vi "Check_Traverse_move.vi"(0 "Current position":dbl[](array[numeric])=[0.0, 0.0, 0.0] format="%.2f", 1 "Traverse Name":string, 2 "Full Check":bool, 5 "New Position":dbl[](array[numeric])=[0.0, 0.0, 0.0] format="%.2f", 7 "Model       Roll      Pitch       Yaw (deg)":dbl[](array[numeric]) format="%#.2f", 9 "Probe Volume":T2=[{"Max"=15.0, "Min"=-15.0}, {"Max"=250.0, "Min"=0.0}, {"Max"=15.0, "Min"=-15.0}] {"Min" format="%#.1f"; "Max" format="%#.1f"}, 11 "Entire Space":T2=[{"Max"=15001.0, "Min"=12000.0}, {"Max"=1000.0, "Min"=-1000.0}, {"Max"=700.0, "Min"=0.0}] {"Min" format="%#.1f"; "Max" format="%#.1f"}, 12 "Exclude Array":T1[](array[typedef])=[{"Sizes"=[{"Max"=15000.0, "Min"=0.0}, {"Max"=1000.0, "Min"=-1000.0}, {"Max"=300.0, "Min"=0.0}], "Name"="Roughness Elements", "Exclude Type"=enum."Allow only vertical moves"}, {"Sizes"=[{"Max"=17000.0, "Min"=16000.0}, {"Max"=200.0, "Min"=-200.0}, {"Max"=-50.0, "Min"=-250.0}], "Name"="B204", "Exclude Type"=enum."Exclude completely"}] {"Sizes"."Min" format="%#.1f"; "Sizes"."Max" format="%#.1f"}) -> (6 "Position At Crash":dbl[](array[numeric]) format="%.2f", 10 "Steps":dbl[][](array[numeric]) format="%.2f", 15 "Error Comments":string)   [LabVIEW 2011]
uses:
  Box_size.ctl
  Exclude_cluster.ctl
  Exclusion_type.ctl
panel:
  # "X                Y                   Z"
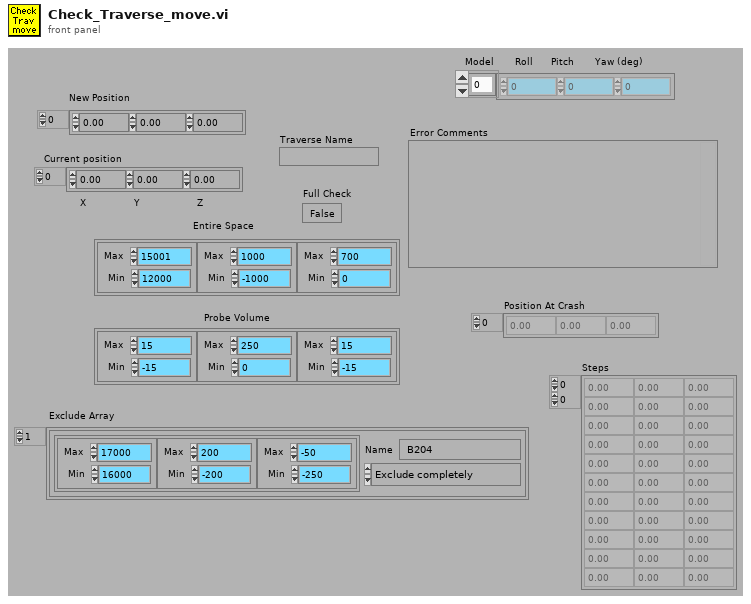
[diagram p1: front panel]
types:
  T1 = typedef "Exclude_cluster.ctl" = cluster{"Sizes":T2, "Name":string, "Exclude Type":T3}
  T2 = typedef "Box_size.ctl" = cluster{"Max":dbl, "Min":dbl}[]
  T3 = typedef "Exclusion_type.ctl" = enum16{"Exclude completely", "Allow only vertical moves"}
  T4 = enum16{"To Traverse Coordinates", "To User Coordinates"}
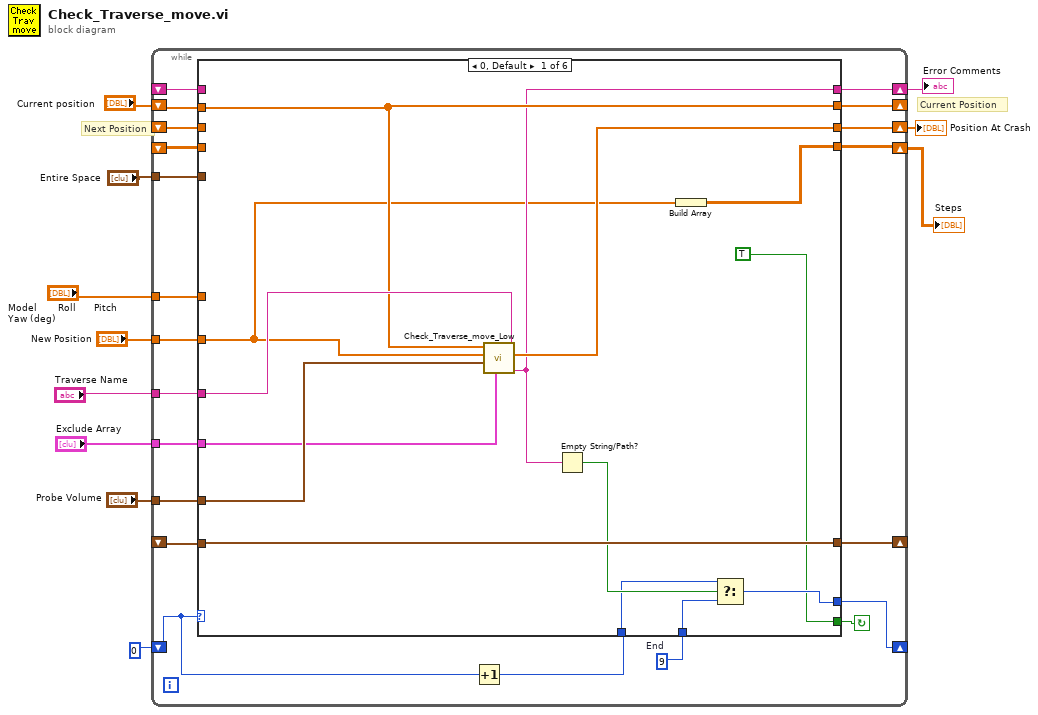
[diagram p0: block diagram]
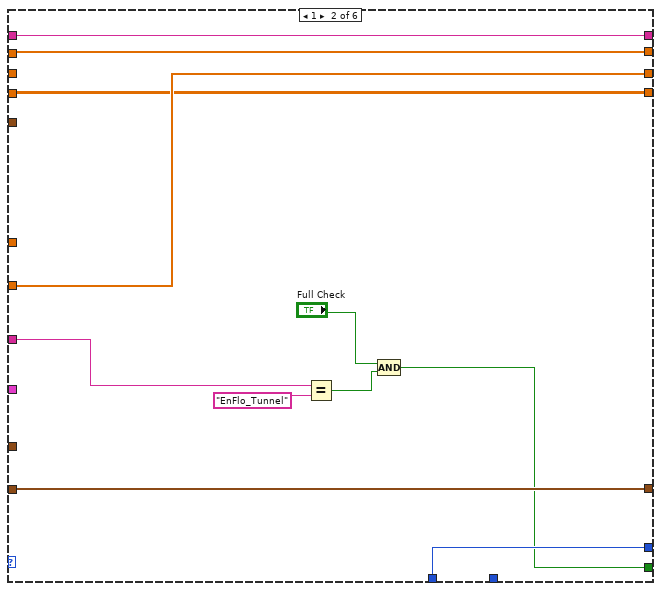
[diagram p2: hidden frame]
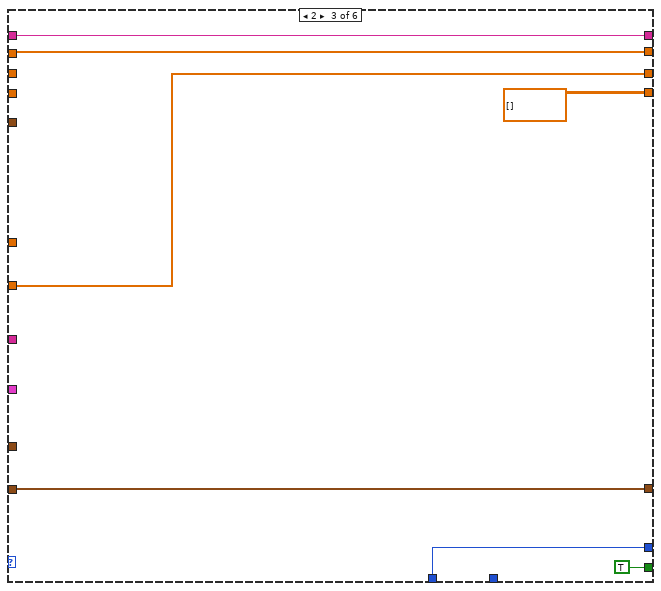
[diagram p3: hidden frame]
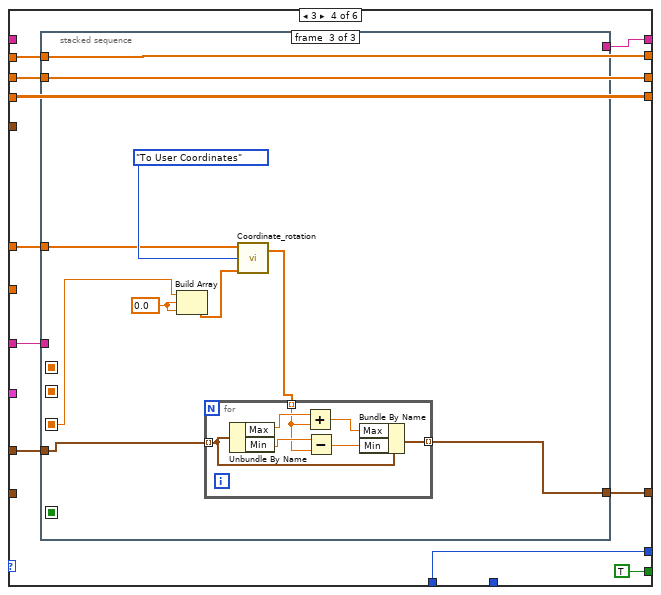
[diagram p4: hidden frame]
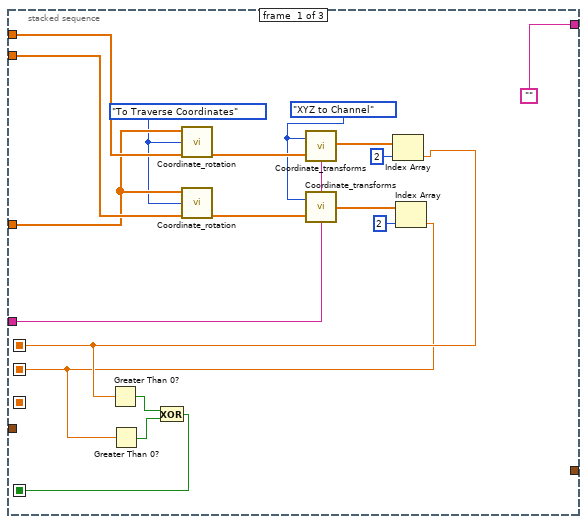
[diagram p5: hidden frame]
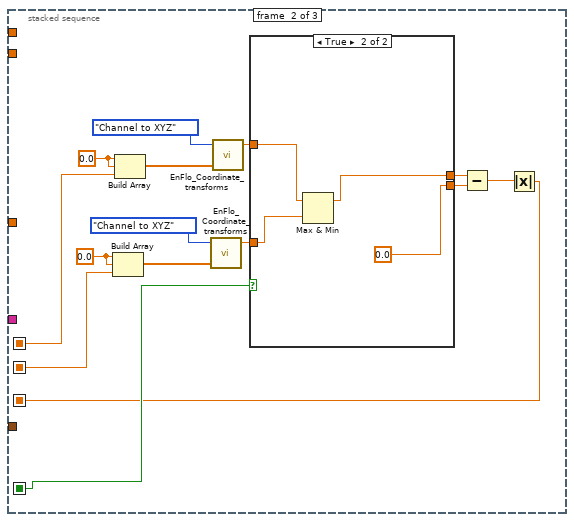
[diagram p6: hidden frame]
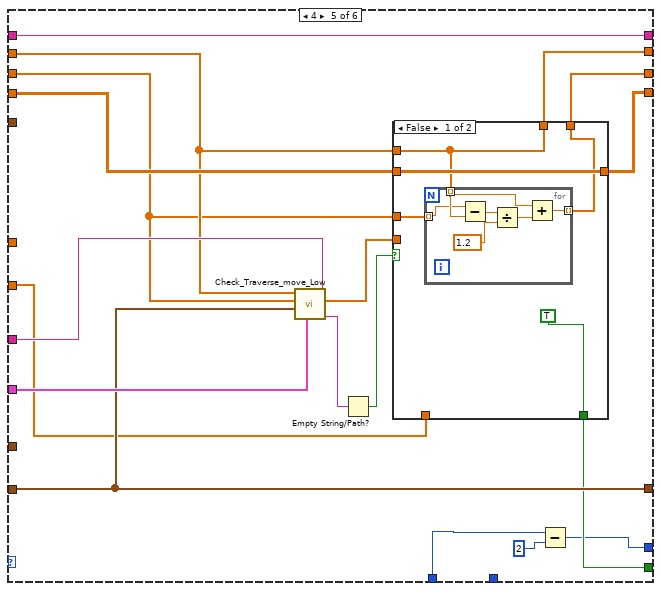
[diagram p8: hidden frame]
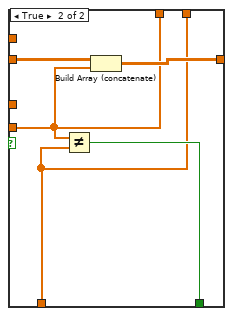
[diagram p9: hidden frame]
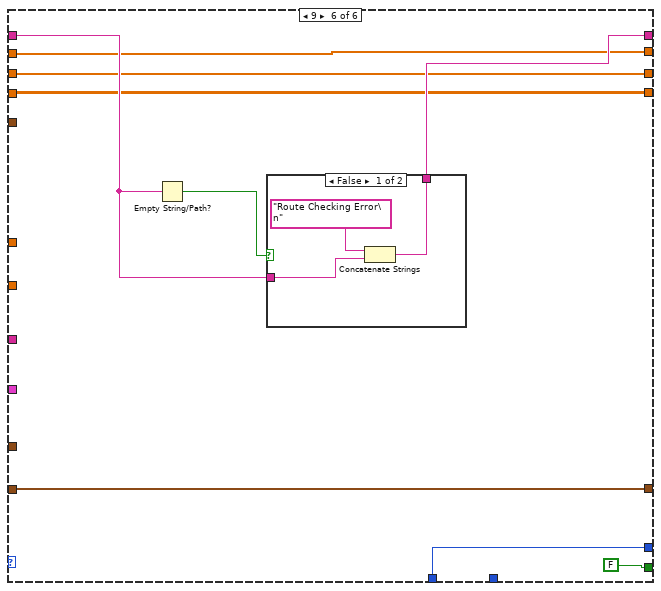
[diagram p10: hidden frame]
diagram:
  # "Current Position"
  # "Next Position"
  n1 = while {
    shift-left: _ -> [w13]
    shift-right: [w12] -> w2
    tunnel: "Probe Volume" -> [w15]
    shift-left: _ -> [w17]
    shift-right: [w16] -> _
    tunnel: "Model       Roll      Pitch       Yaw (deg)" -> [w18]
    tunnel: "New Position" -> [w19]
    shift-left: _ -> [w21]
    shift-right: [w22] -> w6
    shift-left: 0 -> [w25]
    shift-right: [w24] -> _
    tunnel: "Traverse Name" -> [w26]
    tunnel: "Entire Space" -> [w27]
    tunnel: "Exclude Array" -> [w28]
    shift-left: _ -> [w20]
    shift-right: [w30] -> w4
    shift-left: "Current position" -> [w32]
    shift-right: [w31] -> _
    stop <- w29 continue-if-true
    w14 = 9  # End
    n2 = Increment(x=w25) -> (x+1=w23:i32)
    n3 = case shown="0, Default" w25 {
      tunnel: w32 -> [w41 w56 w63 w71 w130 w165]
      tunnel: [w41 w56 w63 w71 w135 w165] -> w31
      tunnel: [w44 w49 w60 w70 w134 w164] -> w30
      tunnel: [TRUE ("Box Inside") w51 TRUE ("Box Inside") TRUE ("Box Inside") w137 FALSE ("Box Inside")] -> w29
      tunnel: w17 -> [w43 w55 w62 _ w144 w166]
      tunnel: w28 -> [w45 _ _ _ w146 _]
      tunnel: w27 -> [_ _ _ _ _ _]
      tunnel: w26 -> [w42 w52 _ w68 w145 _]
      tunnel: [w36 w54 w61 w66 w132 w168] -> w24
      tunnel: w23 -> [w38 w54 w61 w66 w131 w168]
      tunnel: [w40 w57 w64 w74 w142 w169] -> w22
      tunnel: w21 -> [_ w57 w64 _ w142 w170]
      tunnel: w20 -> [_ _ _ w70 w129 w164]
      tunnel: w19 -> [w35 w49 w60 _ w138 _]
      tunnel: w18 -> [_ _ _ w69 _ _]
      tunnel: [w43 w55 w62 w72 w144 w166] -> w16
      tunnel: w15 -> [w46 _ _ w67 _ _]
      tunnel: w14 -> [w37 _ _ _ _ _]
      tunnel: w13 -> [_ w48 _ w65 w141 w163]
      tunnel: [w34 w48 dbl[][] [] w65 w140 w163] -> w12
      frame 0, Default {
        n4 = call "Check_Traverse_move_Low.vi"("Traverse Name"=w42, "Exclude Array"=w45, "Probe Volume"=w46, "New Position"=w35, "Current position"=w41) -> ("Error Comments"=w40:string, "Position At Crash"=w44:dbl[])  [unwired: 1 in, 2 out]
        n5 = Empty String/Path?(string/path=w40) -> (empty?=w39:bool)
        n6 = Build Array(w35) -> (w34:dbl[][])
        n7 = Select(t=w38, s=w39, f=w37) -> (s? t:f=w36:i32)
      }
      frame 1 {
        n8 = Equal?(x=w52, y="EnFlo_Tunnel") -> (x = y?=w47:bool)
        n9 = Compound Arithmetic op=AND("Full Check", w47) -> (w51:bool)
      }
      frame 2 {
      }
      frame 3 {
        n10 = stacked-sequence {
          seq-local: [w77 _ _] -> [_ w107 _]
          seq-local: [w76 _ _] -> [_ w106 _]
          seq-local: [w75 _ _] -> [_ w97 _]
          seq-local: [_ w93 _] -> [_ _ w116]
          tunnel: ["" _ _] -> w74
          tunnel: [_ _ w120] -> w72
          tunnel: w71 -> [w90 _ _]
          tunnel: w70 -> [w88 _ _]
          tunnel: w69 -> [w87 _ w114]
          tunnel: w68 -> [w86 _ _]
          tunnel: w67 -> [_ _ w121]
          frame #0 {
            w84 = enum16{"XYZ to Channel", "Channel to XYZ"}."XYZ to Channel" ("Mode")
            w85 = T4."To Traverse Coordinates" ("Mode")
            n11 = call "Coordinate_rotation.vi"("Model       Roll      Pitch       Yaw (deg)"=w87, "Input Position"=w90, "Mode"=w85) -> ("Output Position"=w91:dbl[])  [unwired: 2 in, 1 out]
            n12 = call "Coordinate_rotation.vi"("Model       Roll      Pitch       Yaw (deg)"=w87, "Input Position"=w88, "Mode"=w85) -> ("Output Position"=w89:dbl[])  [unwired: 2 in, 1 out]
            n13 = call "Coordinate_transforms.vi"("Traverse Name"=w86, "Input"=w91, "Mode"=w84) -> ("Output"=w83:dbl[])
            n14 = call "Coordinate_transforms.vi"("Traverse Name"=w86, "Input"=w89, "Mode"=w84) -> ("Output"=w80:dbl[])
            n15 = Index Array(array=w83, index=2) -> (element=w77:dbl)
            n16 = Greater Than 0?(x=w77) -> (x > 0?=w79:bool)
            n17 = Index Array(array=w80, index=2) -> (element=w76:dbl)
            n18 = Greater Than 0?(x=w76) -> (x > 0?=w78:bool)
            n19 = Exclusive Or(1:w78, 2:w79) -> (0:w75:bool)
          }
          frame #1 {
            w100 = 0.0 ("element")
            w105 = 0.0 ("element")
            n20 = Build Array(w100, w100, w106) -> (w102:dbl[])
            n21 = Build Array(w105, w105, w107) -> (w103:dbl[])
            n22 = call "EnFlo_Coordinate_transforms.vi"("Input"=w102, "Mode"=enum16{"XYZ to Channel", "Channel to XYZ"}."Channel to XYZ") -> ("X theta"=w98:dbl)  [unwired: 3 out]
            n23 = call "EnFlo_Coordinate_transforms.vi"("Input"=w103, "Mode"=enum16{"XYZ to Channel", "Channel to XYZ"}."Channel to XYZ") -> ("X theta"=w99:dbl)  [unwired: 3 out]
            n24 = case shown="True" w97 {
              tunnel: w99 -> [w109 w112]
              tunnel: w98 -> [w108 w113]
              tunnel: [w108 0.0 ("element")] -> w96
              tunnel: [w109 w111] -> w95
              frame False {
              }
              frame True {
                n25 = Max & Min(x=w112, y=w113) -> (max(x,y)=w111:dbl)  [unwired: 1 out]
              }
            }
            n26 = Subtract(x=w95, y=w96) -> (x-y=w94:dbl)
            n27 = Absolute Value(x=w94) -> (abs(x)=w93:dbl)
          }
          frame #2 {
            w118 = 0.0 ("Input Element")
            n28 = Build Array(w116, w118, w118) -> (w117:dbl[])
            n29 = call "Coordinate_rotation.vi"("Model       Roll      Pitch       Yaw (deg)"=w114, "Input Position"=w117, "Mode"=T4."To User Coordinates") -> ("Output Position"=w115:dbl[])  [unwired: 2 in, 1 out]
            n30 = for {
              tunnel: w121 -> [w128] mode=indexing
              tunnel: w115 -> [w123] mode=indexing
              tunnel: [w122] -> w120 mode=indexing
              n31 = Unbundle By Name(w128) -> ("Max"=w127:dbl, "Min"=w126:dbl)
              n32 = Add(x=w127, y=w123) -> (x+y=w125:dbl)
              n33 = Subtract(x=w126, y=w123) -> (x-y=w124:dbl)
              n34 = Bundle By Name(cluster=w128, "Max"=w125, "Min"=w124) -> (w122:cluster{"Max":dbl, "Min":dbl})
            }
          }
        }
      }
      frame 4 {
        n35 = call "Check_Traverse_move_Low.vi"("Traverse Name"=w145, "Exclude Array"=w146, "Probe Volume"=w144, "New Position"=w129, "Current position"=w130) -> ("Error Comments"=w143:string, "Position At Crash"=w136:dbl[])  [unwired: 1 in, 2 out]
        n36 = Empty String/Path?(string/path=w143) -> (empty?=w139:bool)
        n37 = case shown="False" w139 {
          tunnel: w141 -> [w151 w162]
          tunnel: w136 -> [_ w159]
          tunnel: [w151 w161] -> w140
          tunnel: w138 -> [_ w158]
          tunnel: [TRUE w160] -> w137
          tunnel: [w149 w159] -> w135
          tunnel: [w147 w158] -> w134
          tunnel: w130 -> [w149 _]
          tunnel: w129 -> [w148 _]
          frame False {
            n38 = for {
              tunnel: w149 -> [w153] mode=indexing
              tunnel: w148 -> [w152] mode=indexing
              tunnel: [w154] -> w147 mode=indexing
              n39 = Subtract(x=w152, y=w153) -> (x-y=w157:dbl)
              n40 = Divide(x=w157, y=1.2) -> (x/y=w155:dbl)
              n41 = Add(x=w153, y=w155) -> (x+y=w154:dbl)
            }
          }
          frame True {
            n42 = Not Equal?(x=w159, y=w158) -> (x != y?=w160:bool)
            n43 = Build Array (concatenate)(w162, w159) -> (w161:dbl[][])
          }
        }
        n44 = Subtract(x=w131, y=2) -> (x-y=w132:i32)
      }
      frame 9 {
        n45 = Empty String/Path?(string/path=w170) -> (empty?=w171:bool)
        n46 = case shown="False" w171 {
          tunnel: [w172 w175] -> w169
          tunnel: w170 -> [w174 w175]
          frame False {
            n47 = Concatenate Strings("Route Checking Error\n" ("String to match"), w174) -> (w172:string)
          }
          frame True {
          }
        }
      }
    }
  }
  "Error Comments" <- w6
  "Position At Crash" <- w4
  "Steps" <- w2
